vi "Calculate CSP-filter.vi"() -> ()   [LabVIEW 2016]
uses:
  _vlib/CSP.lvclass
  _vlib/CSP_ApplStates.ctl
  Spatial Pattern Filter.lvlib
panel:
  out "Application State":string caption="Текущее состояние"
  in  "Tab Control":enum32{"Инициализация", "Расчет фильтра"}(tab)
  in  "PCA mode":bool
  in  "Start":bool
  in  "NumberOfClasses":i32 caption="Число классов" min=0 max=128 step=1
  out "Class Number":i32 caption="Номер класса"
  out "Processing file":path caption="Обрабатываемый файл"
  out "Label":string caption="Метка класса"
  # "This VI is a part of BCI Design library, http://www.ru-bci.org \nCopyright © 2020, Sotnikov Peter, All rights reserved. License: CC BY-NC 4.0"
  # "Classwise PCA mode"
  # "Вкл."
  # "Обрабатывается класс:"
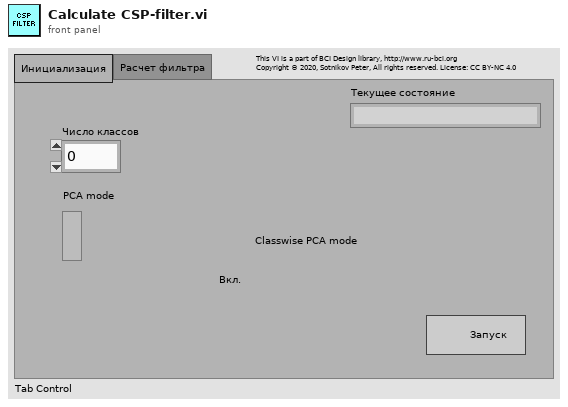
[diagram p1: front panel]
types:
  T1 = typedef "Spatial Pattern Filter.lvlib/CSP_ApplStates.ctl" = enum16{"Initialization", "CalculateCovariance", "CalculateFilter"}
  T2 = cluster{"Class Number":refnum<vi>, "Label":refnum<vi>, "Processing file":refnum<vi>}
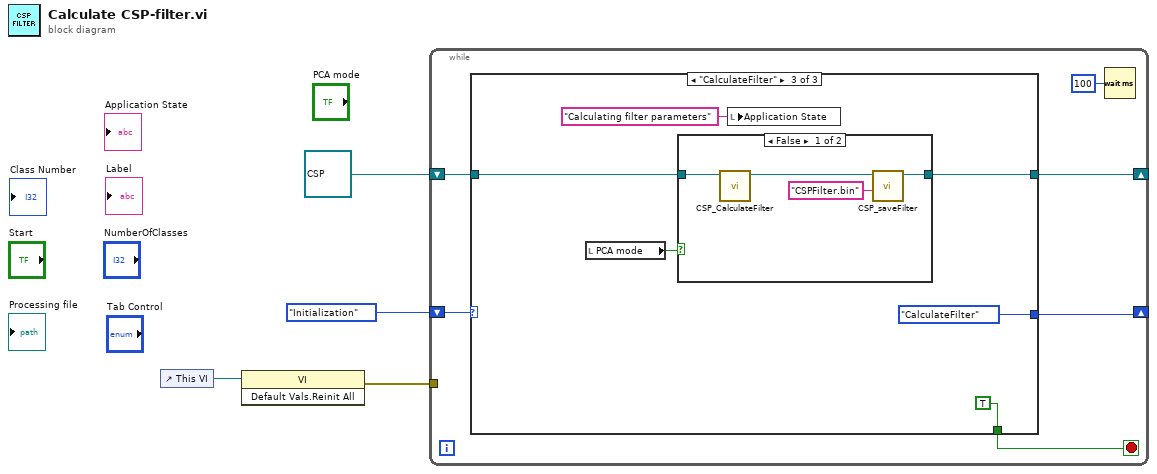
[diagram p0: block diagram]
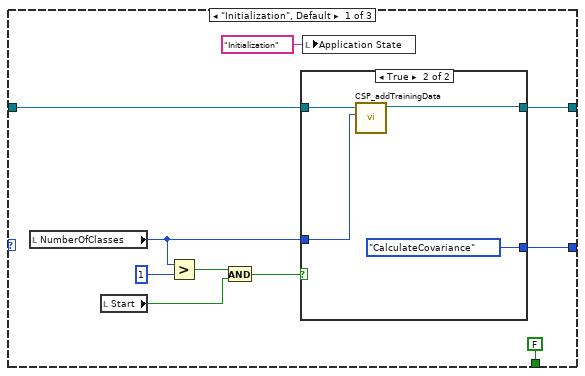
[diagram p2: hidden frame]
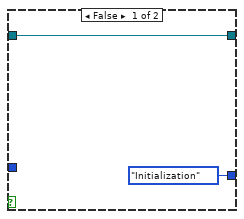
[diagram p3: hidden frame]
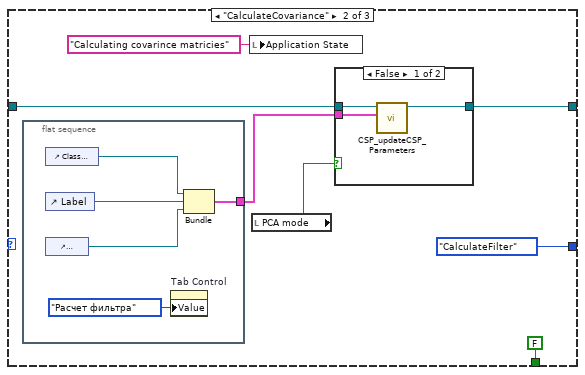
[diagram p4: hidden frame]
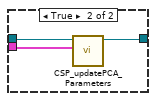
[diagram p5: hidden frame]
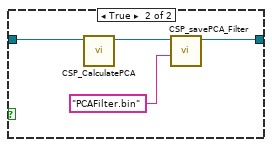
[diagram p6: hidden frame]
diagram:
  n1 = control-ref of="This VI"() -> (w2:refnum<vi>)
  n2 = invoke class="VI" method="Default Vals.Reinit All"(reference=w2) -> (error out=w1:errorcluster)  [unwired: 2 in, 2 out]
  n3 = while {
    shift-right: [w6] -> _
    shift-left: refnum<class "CSP.lvclass"> refnum ("CSP.lvclass") -> [w9]
    shift-right: [w8] -> _
    shift-left: CSP_ApplStates."Initialization" ("ApplicationStates") -> [w10]
    tunnel: w1 -> [_]
    stop <- w5 stop-if-true
    n4 = case shown="\"CalculateFilter\"" w10 {
      tunnel: w9 -> [w17 w32 w48]
      tunnel: [w14 CSP_ApplStates."CalculateFilter" ("ApplicationStates") CSP_ApplStates."CalculateFilter" ("ApplicationStates")] -> w8
      tunnel: [w13 w31 w46] -> w6
      tunnel: [FALSE FALSE TRUE] -> w5
      frame "Initialization", Default {
        n5 = local read "NumberOfClasses"() -> (w16:i32)
        n6 = local read "Start"() -> (w18:bool)
        n7 = Greater?(x=w16, y=1) -> (0:w19:bool)
        n8 = And(x=w19, y=w18) -> (x .and. y?=w15:bool)
        n9 = case shown="True" w15 {
          tunnel: w17 -> [w21 w26]
          tunnel: w16 -> [_ w25]
          tunnel: [CSP_ApplStates."Initialization" ("ApplicationStates") CSP_ApplStates."CalculateCovariance" ("ApplicationStates")] -> w14
          tunnel: [w21 w23] -> w13
          frame False {
          }
          frame True {
            n10 = call "CSP_addTrainingData.vi"("NumberOfClasses"=w25, "CSP.lvclass in"=w26) -> ("CSP.lvclass out"=w23:refnum<class "CSP.lvclass">)  [unwired: 8 in, 1 out]
          }
        }
        n11 = local write "Application State"("Initialization" ("Application State")) -> ()
      }
      frame "CalculateCovariance" {
        n12 = flat-sequence {
          tunnel: [w41] -> w28
          frame #0 {
            n13 = control-ref of="Class Number"() -> (w42:refnum<vi>)
            n14 = control-ref of="Label"() -> (w43:refnum<vi>)
            n15 = control-ref of="Processing file"() -> (w44:refnum<vi>)
            n16 = property on="Tab Control" class="TabCtl (strict)"("Value"=enum32{"Инициализация", "Расчет фильтра"}."Расчет фильтра" ("Tab Control")) -> ()  [unwired: 2 in, 2 out]
            n17 = Bundle("Class Number"=w42, "Label"=w43, "Processing file"=w44) -> (w41:T2)  [unwired: 1 in]
          }
        }
        n18 = local write "Application State"("Calculating covarince matricies" ("Application State")) -> ()
        n19 = local read "PCA mode"() -> (w27:bool)
        n20 = case shown="False" w27 {
          tunnel: w32 -> [w36 w39]
          tunnel: [w35 w37] -> w31
          tunnel: w28 -> [w34 w38]
          frame False {
            n21 = call "CSP_updateCSP_Parameters.vi"("Indicators Ref"=w34, "CSP.lvclass"=w36) -> ("output cluster"=w35:refnum<class "CSP.lvclass">)  [unwired: 8 in, 1 out]
          }
          frame True {
            n22 = call "CSP_updatePCA_Parameters.vi"("Indicators Ref"=w38, "CSP.lvclass in"=w39) -> ("CSP.lvclass out"=w37:refnum<class "CSP.lvclass">)  [unwired: 8 in, 1 out]
          }
        }
      }
      frame "CalculateFilter" {
        n23 = local read "PCA mode"() -> (w45:bool)
        n24 = case shown="False" w45 {
          tunnel: w48 -> [w54 w58]
          tunnel: [w52 w55] -> w46
          frame False {
            n25 = call "CSP_CalculateFilter.vi"("CSP.lvclass"=w54) -> ("CSP.lvclass out"=w53:refnum<class "CSP.lvclass">)  [unwired: 10 in]
            n26 = call "CSP_saveFilter.vi"("File name"="CSPFilter.bin", "CSP.lvclass in"=w53) -> ("CSP.lvclass out"=w52:refnum<class "CSP.lvclass">)  [unwired: 8 in, 1 out]
          }
          frame True {
            n27 = call "CSP_CalculatePCA.vi"("CSP.lvclass in"=w58) -> ("CSP.lvclass out"=w57:refnum<class "CSP.lvclass">)  [unwired: 10 in]
            n28 = call "CSP_savePCA_Filter.vi"("File name"="PCAFilter.bin", "CSP.lvclass in"=w57) -> ("CSP.lvclass out"=w55:refnum<class "CSP.lvclass">)  [unwired: 8 in, 1 out]
          }
        }
        n29 = local write "Application State"("Calculating filter parameters" ("Application State")) -> ()
      }
    }
    n30 = Wait (ms)(milliseconds to wait=u32 100) -> ()  [unwired: 1 out]
  }
